vi "Create Spectrum Writer.vi"(8 "error in (no error)":errorcluster) -> (0 "error out":errorcluster, 3 "Writer":refnum<k21>)   [LabVIEW 2016]
uses:
  <vilib>/dex/Stream Element Allocation Mode.ctl
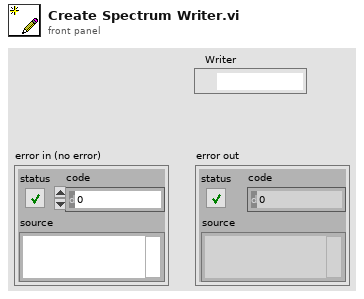
[diagram p1: front panel]
types:
  T1 = typedef "Stream Element Allocation Mode.ctl" = u32
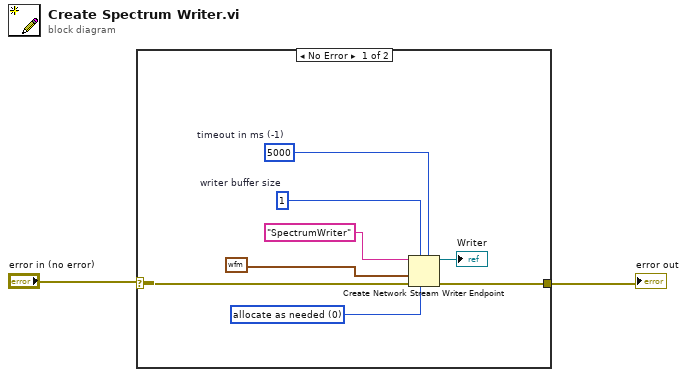
[diagram p0: block diagram]
diagram:
  n1 = case shown="No Error" "error in (no error)" {
    selector: "error in (no error)" -> [w6 w11]
    tunnel: [w5 w11] -> w1
    frame No Error {
      w7 = T1 0 items=["allocate as needed", "pre-allocate"] ("element allocation mode")
      w8 = 5000  # timeout in ms (-1)
      w9 = 1  # writer buffer size
      n2 = Create Network Stream Writer Endpoint(5:w8, 6:w7, 7:w9, 8:w6, 9:waveform(dbl) {"t0"=timestamp(0 s since 1904-01-01), "dt"=1.0, "Y"=[]} ("output waveform"), 11:"SpectrumWriter" ("writer name")) -> (0:w5:errorcluster, 3:→"Writer":refnum<k21>)  [unwired: 1 in]
    }
    frame Error {
    }
  }
  "error out" <- w1
